vi "get item status.vi"(11 "element":T1) -> (2 "Disabled?":bool, 3 "symbol index":i32)   [LabVIEW 2016, in "FPGA Addon System Explorer.lvlib"]
uses:
  FPGA Addon System Explorer.lvlib
  reservation type.ctl
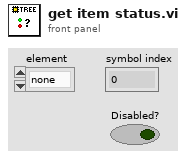
[diagram p1: front panel]
types:
  T1 = typedef "FPGA Addon System Explorer.lvlib/reservation type.ctl" = enum16{"none", "available", "reserved by this", "reserved by other", "incompatible", "parent"}
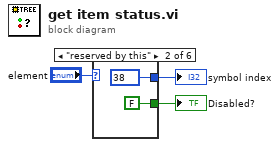
[diagram p0: block diagram]
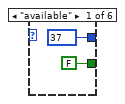
[diagram p2: hidden frame]
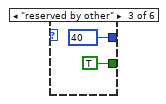
[diagram p3: hidden frame]
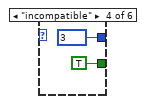
[diagram p4: hidden frame]
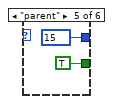
[diagram p5: hidden frame]
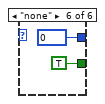
[diagram p6: hidden frame]
diagram:
  n1 = case shown="\"reserved by this\"" "element" {
    tunnel: [37 38 40 3 15 0] -> w2
    tunnel: [FALSE ("Active Item:Disabled?") FALSE ("Active Item:Disabled?") TRUE ("Active Item:Disabled?") TRUE ("Active Item:Disabled?") TRUE ("Active Item:Disabled?") TRUE ("Active Item:Disabled?")] -> w3
    frame "available" {
    }
    frame "reserved by this" {
    }
    frame "reserved by other" {
    }
    frame "incompatible" {
    }
    frame "parent" {
    }
    frame "none" {
    }
  }
  "Disabled?" <- w3
  "symbol index" <- w2
